vi "engine.logger.vi"(6 "isRunning":bool, 8 "Proc Error":errorcluster, 9 "Next State in":cluster{"CMD":T3, "data":variant}={"CMD"=enum."JUMP", "data"=variant}, 10 "Procedure(pre)":variant[](array[variant]), 11 "Procedure(post) in":variant[](array[variant])) -> (0 "error IO":errorcluster, 1 "output cluster":T1 {"clk" format="%#.3f"}, 3 "Procedure out":variant[](array[variant]))   [LabVIEW 2024]
uses:
  controls/typeCmdPostStepFunc.ctl
  controls/type.StepFunction.ctl
  controls/typeEngineLogCluster.ctl
  controls/typeProcVarientName.ctl
  Polymorphics/variantCtrlString.vi
  Polymorphics/variantCtrlNumber.vi
  Polymorphics/variantCtrlStepFunction.vi
  proc.util.validateParamExist.vi
  <vilib>/Utility/error.llb/Clear Errors.vi
  proc.util.enumToStrStepVar.vi
  util.error.create.vi
  Polymorphics/variantCtrlStepName.vi
  Polymorphics/variantCtrlStepUserMessage.vi
panel:
  out "Proc Module":string
  out "Log Msg":string
  out "Proc Path":string
  out "Step Name":string
  out "p1.procName":string
  out "p2.report":string
  out "p2.clk":dbl
  out "p1.index":i32
  out "s1.func":T2
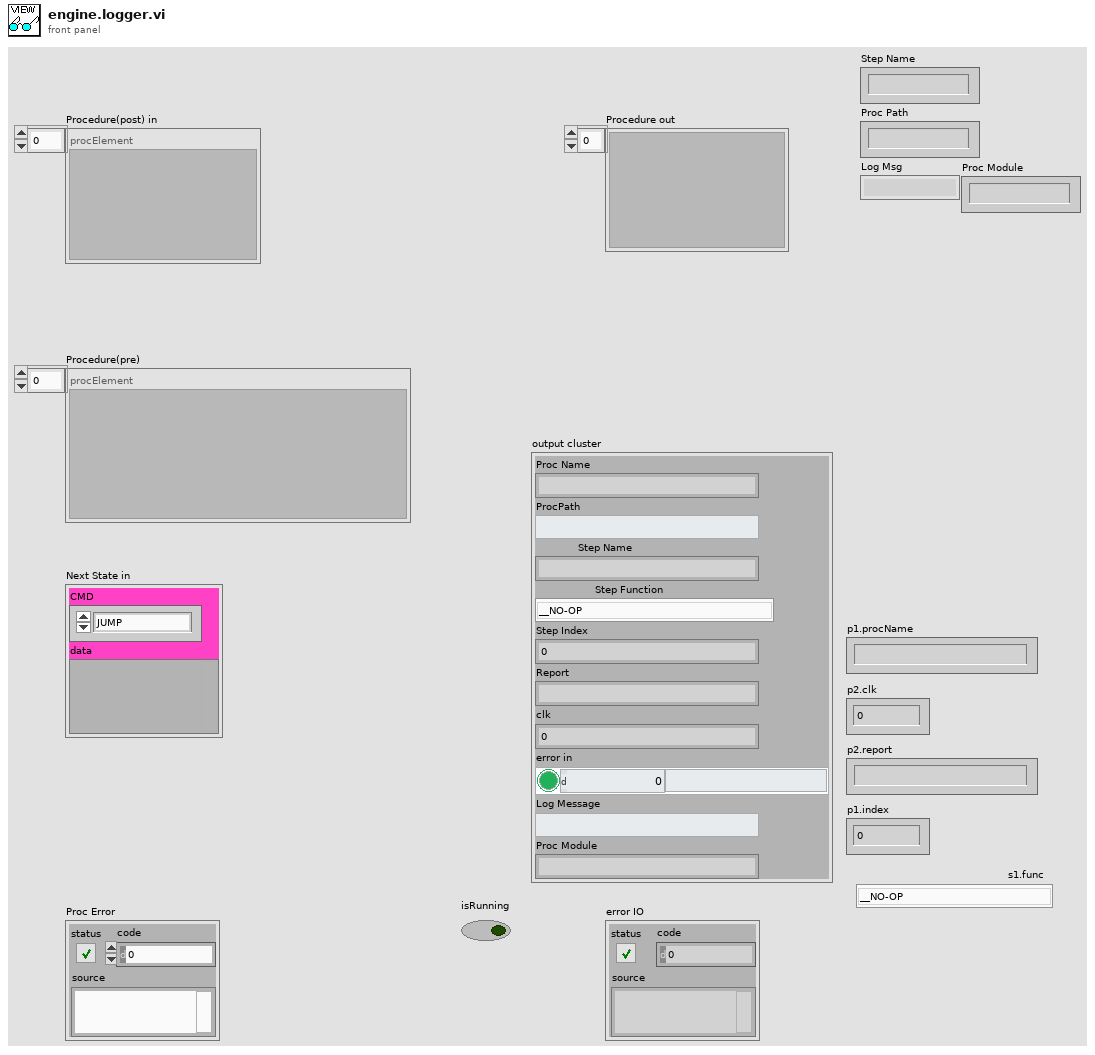
[diagram p1: front panel]
types:
  T1 = typedef "typeEngineLogCluster.ctl" = cluster{"Proc Name":string, "ProcPath":string, "Step Name":string, "Step Function":T2, "Step Index":i32, "Report":string, "clk":dbl, "error in":errorcluster, "Log Message":string, "Proc Module":string}
  T2 = typedef "type.StepFunction.ctl" = enum16{"__NO-OP", "_DELAY_LOAD", "_DELAY_COMPARE", "_JUMP", "_COMPLETE", "_COMPARE", "_LOG_MESSAGE", "_LOG_LAST_REPORT", "_SCHEDULE", "_SCHEDULE_DAILY", "CLK_COMPARE", "PROC_START", "PROC_STOP", "PROC_LOAD", "PROC_COMPLETION_CHECK", "PROC_COMPLETION_LOAD", "_IO_READ", "_IO_READ_MANY", "_IO_WRITE", "_IO_WRITE_BY_REG", "_IO_GET_OUTPUT", "_OCS_CHECK", "_OCS_RECORD", "_GET_RH", "_GET_ACC_UV", "_GET_WD", "_GET_WS", "_REC_DELETE", "_REC_MOVE", "_REC_COPY", "_IRR_CHECK", "UNIT_CHECK", "UNIT_SAMPLE", "UNIT_DOSE"}
  T3 = typedef "typeCmdPostStepFunc.ctl" = enum16{"NEXT", "PREV", "JUMP", "STAY", "COMPLETE", "ENGCALL.PROC.START", "ENGCALL.PROC.STOP", "ENGCALL.PROC.COMPLETION-CHECK", "ENGCALL.PROC.INIT", "ERROR"}
  T4 = typedef "typeProcVarientName.ctl" = enum16{"procNameID", "procModuleID", "procPath", "procIsRunning", "procIndex", "procModule", "procRegisterNumeric", "procRegisterString", "procReport", "procReportPrev", "procCLK", "procStepPointer", "procType"}
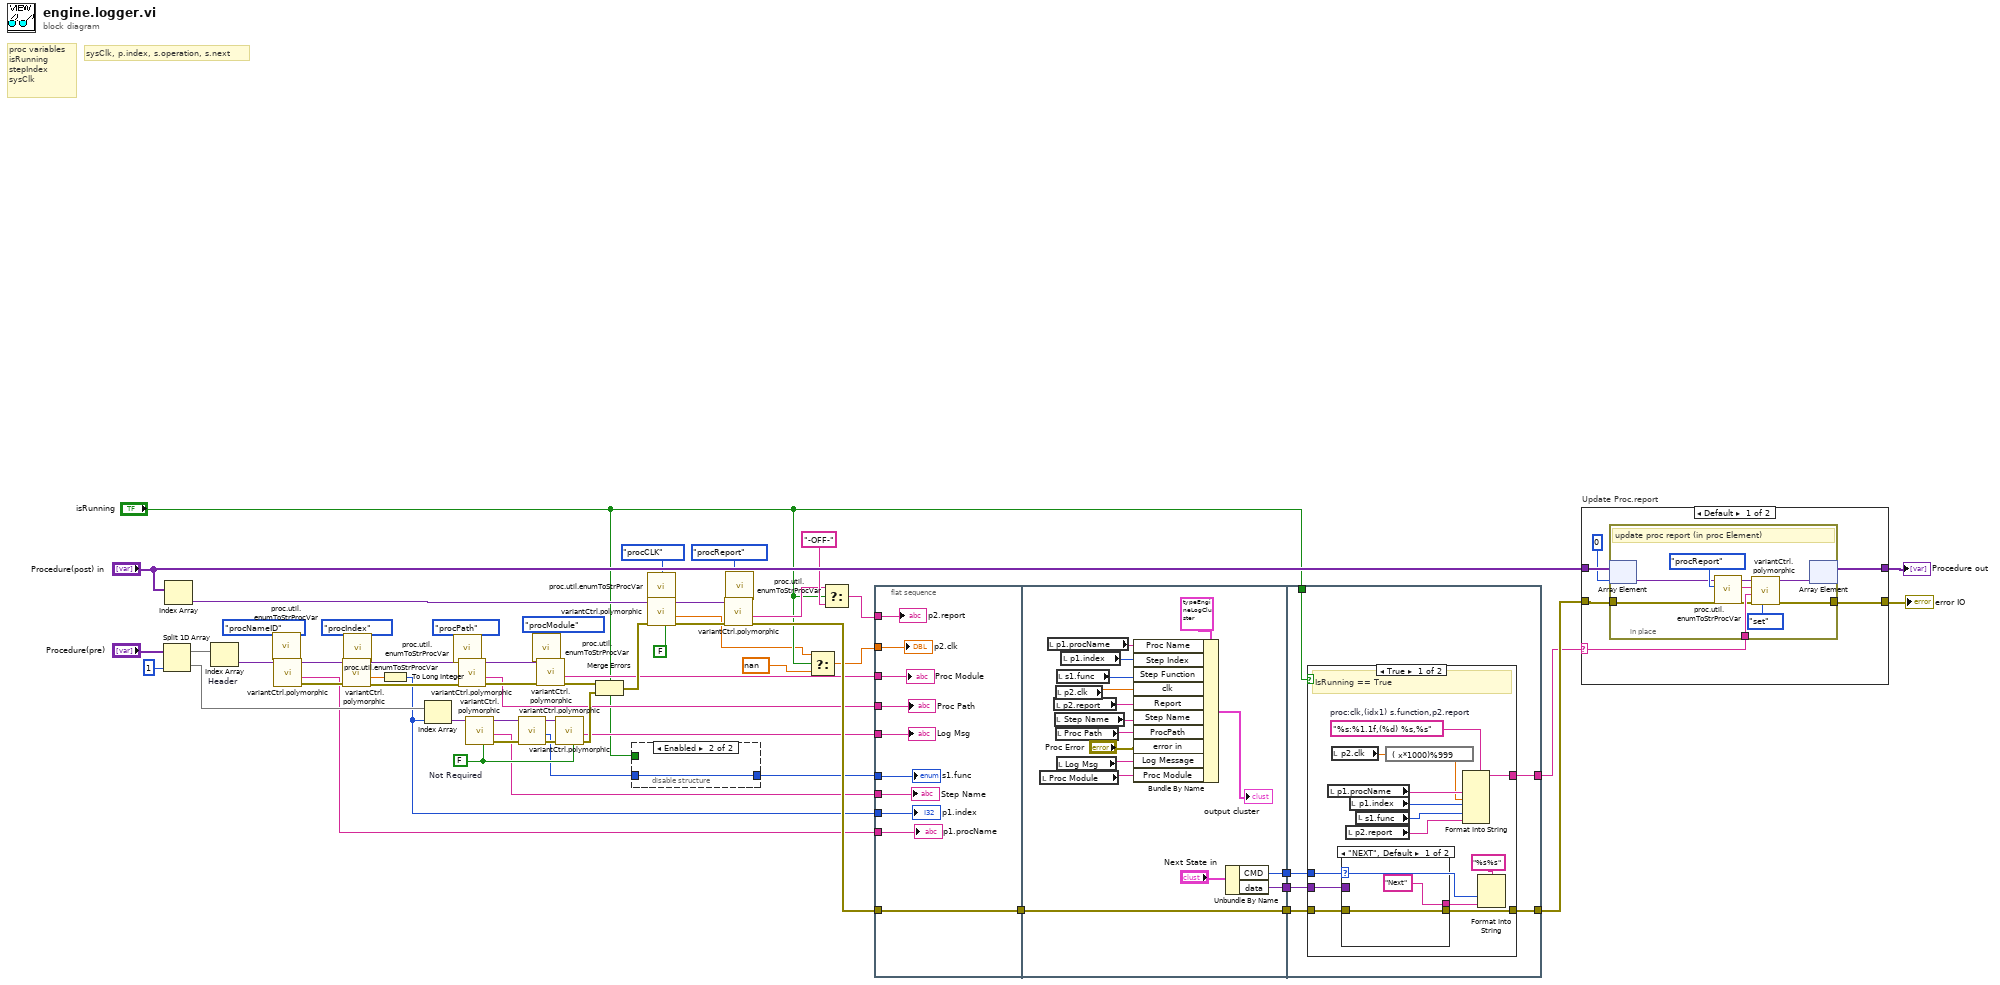
[diagram p0: block diagram]
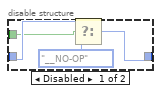
[diagram p2: hidden frame]
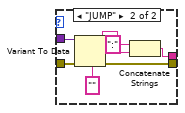
[diagram p3: hidden frame]
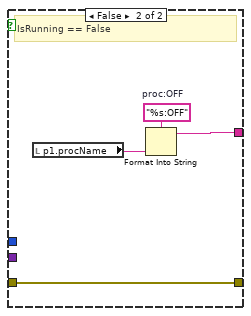
[diagram p4: hidden frame]
diagram:
  w24 = FALSE  # Not Required
  # "proc variables\nisRunning\nstepIndex\nsysClk"
  # "sysClk, p.index, s.operation, s.next"
  n1 = Split 1D Array(array="Procedure(pre)", index=1) -> (first subarray=w48:variant[], second subarray=w47:variant[])
  n2 = Index Array(array="Procedure(post) in") -> (element=w50:variant)  [unwired: 1 in]
  n3 = Index Array "Header"(array=w48) -> (element=w44:variant)  [unwired: 1 in]
  n4 = call "proc.util.enumToStrProcVar.vi"("Proc var"=typeProcVarientName."procNameID" ("Combo Box")) -> ("String"=w41:string)  [unwired: 10 in]
  n5 = call-poly "variantCtrl.polymorphic.vi"("name in"=w41, "Step in"=w44) -> ("error out"=w40:errorcluster, "String Value"=w18:string, "Step out"=w43:variant)  [unwired: 6 in, 1 out]
  n6 = call "proc.util.enumToStrProcVar.vi"("Proc var"=typeProcVarientName."procIndex" ("Combo Box")) -> ("String"=w49:string)  [unwired: 10 in]
  n7 = call-poly "variantCtrl.polymorphic.vi"("error in"=w40, "name in"=w49, "variant in"=w43) -> ("error out"=w32:errorcluster, "number"=w46:dbl, "variant out"=w33:variant)  [unwired: 5 in, 1 out]
  n8 = To Long Integer(number=w46) -> (32bit integer=w19:i32)
  n9 = Index Array(array=w47, index=w19) -> (element=w39:variant)
  n10 = call "proc.util.enumToStrProcVar.vi"("Proc var"=typeProcVarientName."procPath") -> ("String"=w35:string)  [unwired: 10 in]
  n11 = call-poly "variantCtrl.polymorphic.vi"("error in"=w32, "name in"=w35, "Step in"=w33) -> ("error out"=w14:errorcluster, "String Value"=w12:string, "Step out"=w15:variant)  [unwired: 5 in, 1 out]
  n12 = call-poly "variantCtrl.polymorphic.vi"("isRequired (T)"=w24, "stepElement in in"=w39) -> ("error out"=w36:errorcluster, "string out"=w20:string, "stepElement out"=w38:variant)  [unwired: 6 in, 1 out]
  n13 = call-poly "variantCtrl.polymorphic.vi"("error in"=w36, "variant in"=w38) -> ("error out"=w27:errorcluster, "StepFunction"=w9:T2, "variant out"=w26:variant)  [unwired: 6 in, 1 out]
  n14 = call "proc.util.enumToStrProcVar.vi"("Proc var"=typeProcVarientName."procModule") -> ("String"=w16:string)  [unwired: 10 in]
  n15 = call-poly "variantCtrl.polymorphic.vi"("error in"=w14, "name in"=w16, "Step in"=w15) -> ("error out"=w13:errorcluster, "String Value"=w11:string)  [unwired: 5 in, 2 out]
  n16 = call-poly "variantCtrl.polymorphic.vi"("isRequired (T)"=w24, "error in"=w27, "stepElement in in"=w26) -> ("error out"=w31:errorcluster, "string out"=w21:string)  [unwired: 5 in, 2 out]
  n17 = Merge Errors(w13, w31) -> (w23:errorcluster)
  n18 = disable-structure shown="Enabled" {
    disable-tunnel: w9 -> [w65 w67]
    disable-tunnel: [w64 w67] -> w8
    disable-tunnel: "isRunning" -> [w63 _]
    frame Disabled {
      n19 = Select(t=w65, s=w63, f=type.StepFunction."__NO-OP") -> (s? t:f=w64:T2)
    }
    frame Enabled {
    }
  }
  n20 = call "proc.util.enumToStrProcVar.vi"("Proc var"=typeProcVarientName."procCLK" ("Combo Box")) -> ("String"=w54:string)  [unwired: 10 in]
  n21 = call-poly "variantCtrl.polymorphic.vi"("isRequired (T)"=FALSE, "error in"=w23, "name in"=w54, "variant in"=w50) -> ("error out"=w51:errorcluster, "number"=w2:dbl, "variant out"=w55:variant)  [unwired: 4 in, 1 out]
  n22 = call "proc.util.enumToStrProcVar.vi"("Proc var"=typeProcVarientName."procReport" ("Combo Box")) -> ("String"=w53:string)  [unwired: 10 in]
  n23 = call-poly "variantCtrl.polymorphic.vi"("error in"=w51, "name in"=w53, "Step in"=w55) -> ("error out"=w29:errorcluster, "String Value"=w6:string)  [unwired: 5 in, 2 out]
  n24 = Select(t=w2, s="isRunning", f=nan) -> (s? t:f=w1:dbl)
  n25 = Select(t=w6, s="isRunning", f="-OFF-") -> (s? t:f=w5:string)
  n26 = flat-sequence {
    tunnel: w29 -> [w77]
    tunnel: [w77] -> w22
    tunnel: w21 -> [w76]
    tunnel: w20 -> [w75]
    tunnel: w8 -> [w74]
    tunnel: w19 -> [w73]
    tunnel: w18 -> [w72]
    tunnel: w5 -> [w71]
    tunnel: w12 -> [w70]
    tunnel: w11 -> [w69]
    tunnel: w1 -> [w68]
    tunnel: [w93] -> w59
    tunnel: [w92] -> w58
    tunnel: [w89] -> w30
    tunnel: w22 -> [w89]
    tunnel: w59 -> [w97]
    tunnel: w58 -> [w99]
    tunnel: "isRunning" -> [w96]
    tunnel: [w98] -> w25
    tunnel: w30 -> [w95]
    tunnel: [w94] -> w28
    frame #0 {
      "p1.procName" <- w72
      "p1.index" <- w73
      "s1.func" <- w74
      "Step Name" <- w75
      "Log Msg" <- w76
      "p2.report" <- w71
      "Proc Path" <- w70
      "Proc Module" <- w69
      "p2.clk" <- w68
    }
    frame #1 {
      n27 = local read "Proc Module"() -> (w78:string)
      n28 = local read "p1.procName"() -> (w88:string)
      n29 = local read "p2.report"() -> (w84:string)
      n30 = local read "Step Name"() -> (w83:string)
      n31 = local read "p2.clk"() -> (w85:dbl)
      n32 = local read "Proc Path"() -> (w82:string)
      n33 = local read "s1.func"() -> (w86:T2)
      n34 = local read "Log Msg"() -> (w81:string)
      n35 = local read "p1.index"() -> (w87:i32)
      n36 = Bundle By Name(cluster=T1 {"Proc Name"="", "ProcPath"="", "Step Name"="", "Step Function"=enum."__NO-OP", "Step Index"=0, "Report"="", "clk"=0.0, "error in"={"status"=FALSE, "code"=0, "source"=""}, "Log Message"="", "Proc Module"=""}, "Proc Name"=w88, "Step Index"=w87, "Step Function"=w86, "clk"=w85, "Report"=w84, "Step Name"=w83, "ProcPath"=w82, "error in"="Proc Error", "Log Message"=w81, "Proc Module"=w78) -> (→"output cluster":T1)
      n37 = Unbundle By Name("Next State in") -> ("CMD"=w93:T3, "data"=w92:variant)
    }
    frame #2 {
      n38 = case shown="True" w96 {
        tunnel: w99 -> [w111 _]
        tunnel: [w110 w126] -> w98
        tunnel: w97 -> [w108 _]
        tunnel: w95 -> [w101 w123]
        tunnel: [w100 w123] -> w94
        frame True {
          w102 = "%s:%1.1f,(%d) %s,%s"  # proc:clk,(idx1) s.function,p2.report
          # "IsRunning == True"
          n39 = local read "p1.procName"() -> (w106:string)
          n40 = local read "p2.clk"() -> (w104:dbl)
          n41 = case shown="\"NEXT\", Default" w108 {
            tunnel: w111 -> [_ w122]
            tunnel: ["Next" w118] -> w105
            tunnel: w101 -> [w114 w117]
            tunnel: [w114 w116] -> w100
            frame "NEXT", Default {
            }
            frame "JUMP" {
              n42 = Variant To Data(error in=w117, type="", Variant=w122) -> (data=w120:string, error out=w116:errorcluster)
              n43 = Concatenate Strings(":" ("string"), w120) -> (w118:string)
            }
          }
          n44 = local read "p2.report"() -> (w109:string)
          n45 = local read "p1.index"() -> (w113:i32)
          n46 = local read "s1.func"() -> (w112:T2)
          n47 = expression code="( x*1000)%999"(w104) -> (w103:dbl)
          n48 = Format Into String(format string=w102, w106, w103, w113, w112, w109) -> (resulting string=w110:string)  [unwired: 2 in, 1 out]
          n49 = Format Into String(format string="%s%s", w108, w105) -> ()  [unwired: 2 in, 2 out]
        }
        frame False {
          w124 = "%s:OFF"  # proc:OFF
          # "IsRunning == False"
          n50 = local read "p1.procName"() -> (w125:string)
          n51 = Format Into String(format string=w124, w125) -> (resulting string=w126:string)  [unwired: 2 in, 1 out]
        }
      }
    }
  }
  n52 = case "Update Proc.report" shown="Default" w25 {
    selector: w25 -> [w129 _]
    tunnel: [w132 w142] -> w62
    tunnel: "Procedure(post) in" -> [w131 w142]
    tunnel: [w128 w141] -> w60
    tunnel: w28 -> [w127 w141]
    frame Default {
      n53 = in-place {
        in-place-border: w129 -> [w136]
        in-place-border: [w134] -> w128
        in-place-border: w127 -> [w133]
        # "update proc report (in proc Element)"
        n54 = in-place-array #1(w131, 0) -> (w138:variant)
        n55 = call "proc.util.enumToStrProcVar.vi"("Proc var"=typeProcVarientName."procReport") -> ("String"=w140:string)  [unwired: 10 in]
        n56 = call-poly "variantCtrl.polymorphic.vi"("menu in (get)"=enum16{"get", "set"}."set", "error in"=w133, "String Value"=w136, "name in"=w140, "Step in"=w138) -> ("error out"=w134:errorcluster, "Step out"=w137:variant)  [unwired: 3 in, 2 out]
        n57 = in-place-array #1(w137) -> (w132:variant[])  [unwired: 1 out]
      }
    }
    frame "" {
    }
  }
  "error IO" <- w60
  "Procedure out" <- w62
